vi "DSF.Execution.Builder.Command.Send.vi"(8 "error in (no error)":errorcluster, 9 "timeout in ms (0)":i32, 10 "Command":T1={"Command"=enum."Build", "Plugin ID"=0, "Transfer ID"=0}, 11 "Builder in":refnum<class "DSF.Execution.Builder.lvclass">) -> (0 "error out":errorcluster, 1 "timed out?":bool, 3 "Builder out":refnum<class "DSF.Execution.Builder.lvclass">)   [LabVIEW 2016, in "DSF.Engine.lvlib" / "DSF.Execution.Builder.lvclass"]
uses:
  DSF.Execution.Builder.lvclass
  DSF.Execution.Builder.Command Payload.ctl
  DSF.Execution.Builder.Commands.ctl
  DSF.Execution.Builder.lvclass/DSF.Execution.Builder.ctl
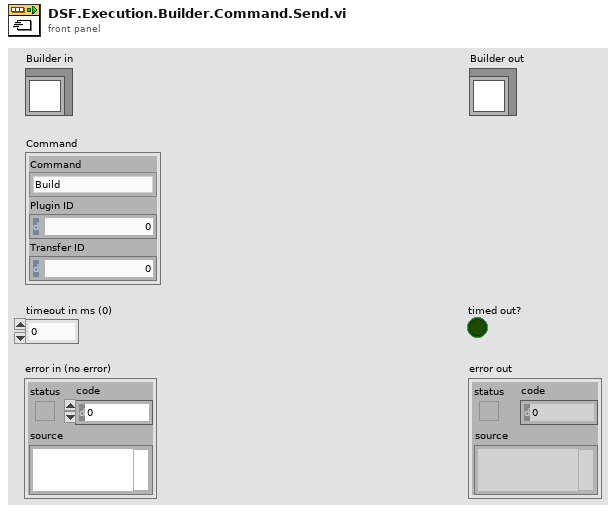
[diagram p1: front panel]
types:
  T1 = typedef "DSF.Engine.lvlib/DSF.Execution.Builder.lvclass/DSF.Execution.Builder.Command Payload.ctl" = cluster{"Command":T2, "Plugin ID":i32, "Transfer ID":i32}
  T2 = typedef "DSF.Engine.lvlib/DSF.Execution.Builder.lvclass/DSF.Execution.Builder.Commands.ctl" = enum8{"Initialize", "Build", "Parse", "Shutdown"}
  T3 = typedef "DSF.Engine.lvlib/DSF.Execution.Builder.lvclass/DSF.Execution.Builder.FIFOs.ctl" = cluster{"Command FIFO":T4, "Response FIFO":T5}
  T4 = typedef "DSF.Engine.lvlib/DSF.Execution.Builder.lvclass/DSF.Execution.Builder.Command FIFO.ctl" = refnum<k33>
  T5 = typedef "DSF.Engine.lvlib/DSF.Execution.Builder.lvclass/DSF.Execution.Builder.Response FIFO.ctl" = refnum<k33>
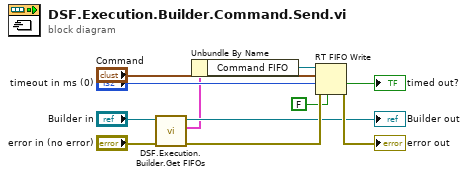
[diagram p0: block diagram]
diagram:
  n1 = call "DSF.Execution.Builder.Get FIFOs.vi"("error in (no error)"="error in (no error)", "Builder in"="Builder in") -> ("error out"=w8:errorcluster, "FIFOs"=w1:T3, "Builder out"=→"Builder out":refnum<class "DSF.Execution.Builder.lvclass">)  [unwired: 7 in]
  n2 = Unbundle By Name(w1) -> ("Command FIFO"=w9:T4)
  n3 = RT FIFO Write(0:w9, 1:"Command", 2:"timeout in ms (0)", 3:w8, 5:FALSE ("overwrite on timeout (T)")) -> (10:→"timed out?":bool, 11:→"error out":errorcluster)  [unwired: 2 out]
